vi "IMAQ FPGA CXP Wait For EOI.vi"(10 "EOI":bool, 11 "Reset":bool) -> (3 "Enable":bool)   [LabVIEW 2020]
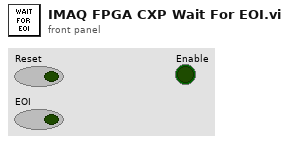
[diagram p1: front panel]
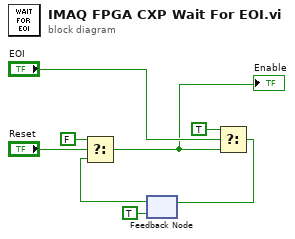
[diagram p0: block diagram]
diagram:
  n1 = feedback #1(TRUE ("f")) -> (w6:bool)
  n2 = Select(t=FALSE, s="Reset", f=w6) -> (s? t:f=w1:bool)
  "Enable" <- w1
  n3 = Select(t=TRUE ("f"), s="EOI", f=w1) -> (s? t:f=w5:bool)
  n4 = feedback-in #1(w5) -> ()
